vi "SetCString_byPtr.vi"(4 "error in (no error)":errorcluster, 6 "Input":string, 7 "Pointer":i32) -> (0 "error out":errorcluster, 3 "Duplicate Pointer":i32)   [LabVIEW 2011]
doc: "Use this VI to se the value of any C String (NULL terminated) in memory. \n\n*Warning- The pointer VIs access memory directly. The VIs check for NULL pointers but may still cause access violations and crashes if used to access protected or otherwise inaccessible memory locations."
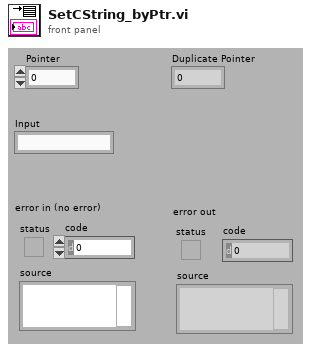
[diagram p1: front panel]
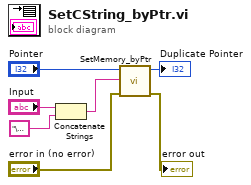
[diagram p0: block diagram]
diagram:
  n1 = Concatenate Strings("Input", "\u0000" ("string")) -> (w4:string)
  n2 = call "SetMemory_byPtr.vi"("error in (no error)"="error in (no error)", "Input"=w4, "Pointer"="Pointer") -> ("error out"=→"error out":errorcluster, "Duplicate Pointer"=→"Duplicate Pointer":i32)  [unwired: 4 out]
